vi "PWM Wing Duty Cycle Calculation.vi"(9 "End Angle Duty Cycle":fxp<+,8,0>, 10 "Start Angle Duty Cycle":fxp<+,8,0>, 11 "Sector":u8) -> (3 "Duty Cycle Out":fxp<+/-,9,1>)   [LabVIEW 2013]
uses:
  <vilib>/rvi/Analysis/common/FxpNativeNode/niFpgaFxpNative.xnode
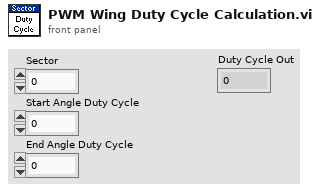
[diagram p1: front panel]
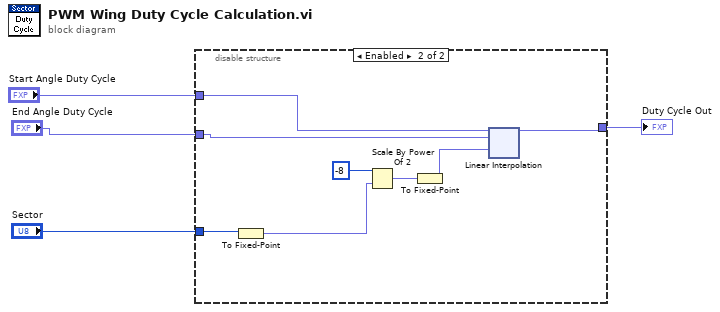
[diagram p0: block diagram]
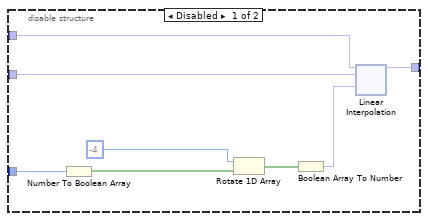
[diagram p2: hidden frame]
diagram:
  n1 = disable-structure shown="Enabled" {
    disable-tunnel: "Start Angle Duty Cycle" -> [w12 w26]
    disable-tunnel: "End Angle Duty Cycle" -> [w11 w25]
    disable-tunnel: [w10 w24] -> w2
    disable-tunnel: "Sector" -> [w9 w28]
    frame Disabled {
      n2 = Number To Boolean Array(number=w9) -> (Boolean array=w8:bool[])
      n3 = Rotate 1D Array(1:w8, 2:-4 ("n")) -> (0:w7:bool[])
      n4 = Boolean Array To Number(Boolean array=w7) -> (number=w6:fxp<+,8,0>)
      n5 = xnode ("Linear Interpolation")("y0"=w12, "y1"=w11, "x"=w6) -> ("y"=w10:fxp<+/-,9,1>)
    }
    frame Enabled {
      n6 = To Fixed-Point(number=w28) -> (fixed-point=w27:fxp<+,32,8>)  [unwired: 1 in]
      n7 = Scale By Power Of 2(n=i16 -8, x=w27) -> (x*2^n=w30:fxp<+,32,8>)
      n8 = To Fixed-Point(number=w30) -> (fixed-point=w31:fxp<+,8,0>)  [unwired: 1 in]
      n9 = xnode ("Linear Interpolation")("y0"=w26, "y1"=w25, "x"=w31) -> ("y"=w24:fxp<+/-,9,1>)
    }
  }
  "Duty Cycle Out" <- w2
